vi "svx_Oct_Waterfall Init.vi"(3 "Container State":T5, 4 "Previous State":variant=variant(cluster{"X Scale Width %":dbl, "Y Scale Height %":dbl, "X-Axis Range":cluster{"Minimum":dbl, "Maximum":dbl}, "Y-Axis Range":cluster{"Minimum":dbl, "Maximum":dbl}, "Z-Axis Range":cluster{"Minimum":dbl, "Maximum":dbl}, "# Plots Updated":i32, "Plot Color":u32, "Frame Color":u32, "Background Color":u32, "Property Name":string, "Just Loaded?":bool, "Initial AutoScale Y":bool, "AutoScale X":u8, "AutoScale Y":u8, "AutoScale Z":u8, "Plot Transparency":bool, "X-Axis Name":string, "Y-Axis Name":string, "Z-Axis Name":string, "X-Axis Scaling Factor":cluster{"Offset":dbl, "Multiplier":dbl}, "Y-Axis Scaling Factor":cluster{"Offset":dbl, "Multiplier":dbl}, "Z-Axis Scaling Factor":cluster{"Offset":dbl, "Multiplier":dbl}, "X-Scale Visible":bool, "Y-Scale Visible":bool, "Z-Scale Visible":bool, "X-Scale Label Visible":bool, "Y-Scale Label Visible":bool, "Z-Scale Label Visible":bool, "X-Axis Range Scaled":cluster{"Minimum":dbl, "Maximum":dbl}, "Y-Axis Range Scaled":cluster{"Minimum":dbl, "Maximum":dbl}, "Z-Axis Range Scaled":cluster{"Minimum":dbl, "Maximum":dbl}, "Rev Z Order":bool, "First Time Ever":bool} {"X Scale Width %"=0.0, "Y Scale Height %"=0.0, "X-Axis Range"={"Minimum"=0.0, "Maximum"=0.0}, "Y-Axis Range"={"Minimum"=0.0, "Maximum"=0.0}, "Z-Axis Range"={"Minimum"=0.0, "Maximum"=0.0}, "# Plots Updated"=0, "Plot Color"=0, "Frame Color"=0, "Background Color"=0, "Property Name"="", "Just Loaded?"=FALSE, "Initial AutoScale Y"=FALSE, "AutoScale X"=0, "AutoScale Y"=0, "AutoScale Z"=0, "Plot Transparency"=FALSE, "X-Axis Name"="", "Y-Axis Name"="", "Z-Axis Name"="", "X-Axis Scaling Factor"={"Offset"=0.0, "Multiplier"=0.0}, "Y-Axis Scaling Factor"={"Offset"=0.0, "Multiplier"=0.0}, "Z-Axis Scaling Factor"={"Offset"=0.0, "Multiplier"=0.0}, "X-Scale Visible"=FALSE, "Y-Scale Visible"=FALSE, "Z-Scale Visible"=FALSE, "X-Scale Label Visible"=FALSE, "Y-Scale Label Visible"=FALSE, "Z-Scale Label Visible"=FALSE, "X-Axis Range Scaled"={"Minimum"=0.0, "Maximum"=0.0}, "Y-Axis Range Scaled"={"Minimum"=0.0, "Maximum"=0.0}, "Z-Axis Range Scaled"={"Minimum"=0.0, "Maximum"=0.0}, "Rev Z Order"=FALSE, "First Time Ever"=FALSE}), 5 "Previous Version":T4) -> (2 "Current State":T3={"X Scale Width %"=50.0, "Y Scale Height %"=50.0, "X-Axis Range"={"Minimum"=0.0, "Maximum"=10.0}, "Y-Axis Range"={"Minimum"=0.0, "Maximum"=10.0}, "Z-Axis Range"={"Minimum"=0.0, "Maximum"=10.0}, "Plot Color"=0, "Frame Color"=61212, "Background Color"=16252785, "Initial AutoScale Y"=TRUE, "AutoScale X"=2, "AutoScale Y"=2, "AutoScale Z"=2, "Plot Transparency"=FALSE, "X-Axis Name"="Frequency", "Y-Axis Name"="Amplitude", "Z-Axis Name"="", "X-Axis Scaling Factor"={"Offset"=0.0, "Multiplier"=1.0}, "Y-Axis Scaling Factor"={"Offset"=0.0, "Multiplier"=1.0}, "Z-Axis Scaling Factor"={"Offset"=0.0, "Multiplier"=1.0}, "X-Scale Visible"=TRUE, "Y-Scale Visible"=TRUE, "Z-Scale Visible"=TRUE, "X-Scale Label Visible"=TRUE, "Y-Scale Label Visible"=TRUE, "Z-Scale Label Visible"=TRUE, "X-Axis Range Scaled"={"Minimum"=0.0, "Maximum"=10.0}, "Y-Axis Range Scaled"={"Minimum"=0.0, "Maximum"=10.0}, "Z-Axis Range Scaled"={"Minimum"=0.0, "Maximum"=10.0}, "Rev Z Order"=FALSE, "X-Scale Format Str"="%#.4g", "Y-Scale Format Str"="%#.4g", "Z-Scale Format Str"="%#.4g", "Decor color"=12369084, "Scale Range Change"=refnum, "out of state queue"=refnum, "property nodes"=refnum})   [LabVIEW 2017, in "SVX Octave Waterfall Graph.xctl"]
uses:
  <vilib>/addons/_XControls/Octave Waterfall Graph/SVX Octave Waterfall Graph.xctl
  <vilib>/addons/_XControls/Octave Waterfall Graph/subVIs/svx_Oct_Waterfall State.ctl
  <vilib>/_xctls/Container State.ctl
  <vilib>/_xctls/Version.ctl
  <vilib>/_xctls/XControlSupport.lvlib
panel:
  out "background":bool
  in  "Indicator State (6.0.0.0, 7.0.0.0)":T1={"X Scale Width %"=80.0, "Y Scale Height %"=40.0, "X-Axis Range"={"Minimum"=0.0, "Maximum"=10.0}, "Y-Axis Range"={"Minimum"=0.0, "Maximum"=10.0}, "Z-Axis Range"={"Minimum"=0.0, "Maximum"=10.0}, "# Plots Updated"=0, "Plot Color"=61212, "Frame Color"=16252785, "Background Color"=16777222, "Property Name"=[], "Just Loaded?"=TRUE, "Initial AutoScale Y"=TRUE, "AutoScale X"=2, "AutoScale Y"=2, "AutoScale Z"=2, "Plot Transparency"=FALSE, "X-Axis Name"="Frequency", "Y-Axis Name"="Amplitude", "Z-Axis Name"="", "X-Axis Scaling Factor"={"Offset"=0.0, "Multiplier"=1.0}, "Y-Axis Scaling Factor"={"Offset"=0.0, "Multiplier"=1.0}, "Z-Axis Scaling Factor"={"Offset"=0.0, "Multiplier"=1.0}, "X-Scale Visible"=TRUE, "Y-Scale Visible"=TRUE, "Z-Scale Visible"=TRUE, "X-Scale Label Visible"=TRUE, "Y-Scale Label Visible"=TRUE, "Z-Scale Label Visible"=TRUE, "X-Axis Range Scaled"={"Minimum"=0.0, "Maximum"=10.0}, "Y-Axis Range Scaled"={"Minimum"=0.0, "Maximum"=10.0}, "Z-Axis Range Scaled"={"Minimum"=0.0, "Maximum"=10.0}, "Rev Z Order"=FALSE, "First Time Ever"=TRUE, "X-Scale Format Str"="%#.4g", "Y-Scale Format Str"="%#.4g", "Z-Scale Format Str"="%#.4g", "Decor color"=12369084, "Facade VI"=refnum, "Scale Range Change"=refnum}
  in  "Indicator State (5.0.0.0)":T2={"X Scale Width %"=80.0, "Y Scale Height %"=40.0, "X-Axis Range"={"Minimum"=0.0, "Maximum"=10.0}, "Y-Axis Range"={"Minimum"=0.0, "Maximum"=10.0}, "Z-Axis Range"={"Minimum"=0.0, "Maximum"=10.0}, "# Plots Updated"=0, "Plot Color"=61212, "Frame Color"=16252785, "Background Color"=16777222, "Property Name"=[], "Just Loaded?"=TRUE, "Initial AutoScale Y"=TRUE, "AutoScale X"=2, "AutoScale Y"=2, "AutoScale Z"=2, "Plot Transparency"=FALSE, "X-Axis Name"="Frequency", "Y-Axis Name"="Amplitude", "Z-Axis Name"="", "X-Axis Scaling Factor"={"Offset"=0.0, "Multiplier"=1.0}, "Y-Axis Scaling Factor"={"Offset"=0.0, "Multiplier"=1.0}, "Z-Axis Scaling Factor"={"Offset"=0.0, "Multiplier"=1.0}, "X-Scale Visible"=TRUE, "Y-Scale Visible"=TRUE, "Z-Scale Visible"=TRUE, "X-Scale Label Visible"=TRUE, "Y-Scale Label Visible"=TRUE, "Z-Scale Label Visible"=TRUE, "X-Axis Range Scaled"={"Minimum"=0.0, "Maximum"=10.0}, "Y-Axis Range Scaled"={"Minimum"=0.0, "Maximum"=10.0}, "Z-Axis Range Scaled"={"Minimum"=0.0, "Maximum"=10.0}, "Rev Z Order"=FALSE, "First Time Ever"=TRUE, "X-Scale Format Str"="%#.4g", "Y-Scale Format Str"="%#.4g", "Z-Scale Format Str"="%#.4g", "Decor color"=12369084, "Facade VI"=refnum}
  in  "Default Indicator State":T3={"X Scale Width %"=80.0, "Y Scale Height %"=40.0, "X-Axis Range"={"Minimum"=0.0, "Maximum"=10.0}, "Y-Axis Range"={"Minimum"=0.0, "Maximum"=10.0}, "Z-Axis Range"={"Minimum"=0.0, "Maximum"=10.0}, "Plot Color"=6618880, "Frame Color"=16252785, "Background Color"=16777222, "Initial AutoScale Y"=TRUE, "AutoScale X"=2, "AutoScale Y"=2, "AutoScale Z"=2, "Plot Transparency"=FALSE, "X-Axis Name"="Frequency", "Y-Axis Name"="Amplitude", "Z-Axis Name"="", "X-Axis Scaling Factor"={"Offset"=0.0, "Multiplier"=1.0}, "Y-Axis Scaling Factor"={"Offset"=0.0, "Multiplier"=1.0}, "Z-Axis Scaling Factor"={"Offset"=0.0, "Multiplier"=1.0}, "X-Scale Visible"=TRUE, "Y-Scale Visible"=TRUE, "Z-Scale Visible"=TRUE, "X-Scale Label Visible"=TRUE, "Y-Scale Label Visible"=TRUE, "Z-Scale Label Visible"=TRUE, "X-Axis Range Scaled"={"Minimum"=0.0, "Maximum"=10.0}, "Y-Axis Range Scaled"={"Minimum"=0.0, "Maximum"=10.0}, "Z-Axis Range Scaled"={"Minimum"=0.0, "Maximum"=10.0}, "Rev Z Order"=FALSE, "X-Scale Format Str"="%#.4g", "Y-Scale Format Str"="%#.4g", "Z-Scale Format Str"="%#.4g", "Decor color"=12369084, "Scale Range Change"=refnum, "out of state queue"=refnum, "property nodes"=refnum}
  in  "Default Control State":T3={"X Scale Width %"=80.0, "Y Scale Height %"=40.0, "X-Axis Range"={"Minimum"=0.0, "Maximum"=10.0}, "Y-Axis Range"={"Minimum"=0.0, "Maximum"=10.0}, "Z-Axis Range"={"Minimum"=0.0, "Maximum"=10.0}, "Plot Color"=6618880, "Frame Color"=16252785, "Background Color"=16777222, "Initial AutoScale Y"=TRUE, "AutoScale X"=2, "AutoScale Y"=2, "AutoScale Z"=2, "Plot Transparency"=FALSE, "X-Axis Name"="Frequency", "Y-Axis Name"="Amplitude", "Z-Axis Name"="", "X-Axis Scaling Factor"={"Offset"=0.0, "Multiplier"=1.0}, "Y-Axis Scaling Factor"={"Offset"=0.0, "Multiplier"=1.0}, "Z-Axis Scaling Factor"={"Offset"=0.0, "Multiplier"=1.0}, "X-Scale Visible"=TRUE, "Y-Scale Visible"=TRUE, "Z-Scale Visible"=TRUE, "X-Scale Label Visible"=TRUE, "Y-Scale Label Visible"=TRUE, "Z-Scale Label Visible"=TRUE, "X-Axis Range Scaled"={"Minimum"=0.0, "Maximum"=10.0}, "Y-Axis Range Scaled"={"Minimum"=0.0, "Maximum"=10.0}, "Z-Axis Range Scaled"={"Minimum"=0.0, "Maximum"=10.0}, "Rev Z Order"=FALSE, "X-Scale Format Str"="%#.4g", "Y-Scale Format Str"="%#.4g", "Z-Scale Format Str"="%#.4g", "Decor color"=12369084, "Scale Range Change"=refnum, "out of state queue"=refnum, "property nodes"=refnum}
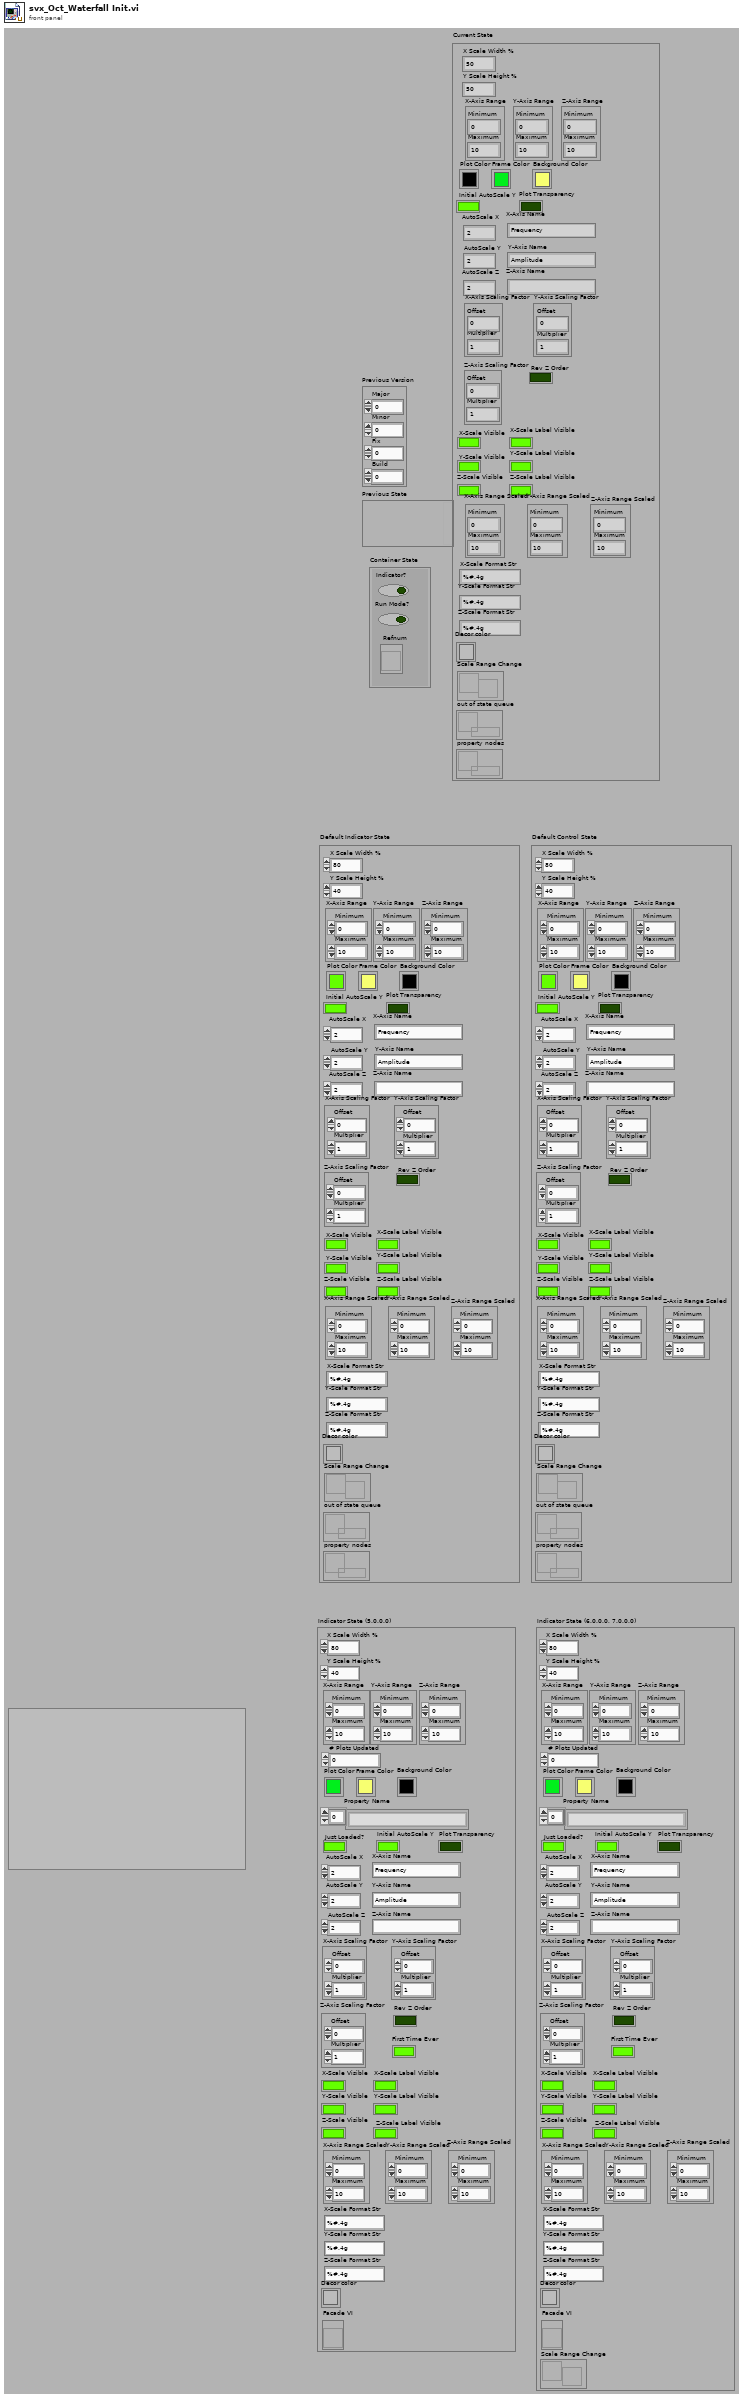
[diagram p1: front panel]
types:
  T1 = cluster{"X Scale Width %":dbl, "Y Scale Height %":dbl, "X-Axis Range":cluster{"Minimum":dbl, "Maximum":dbl}, "Y-Axis Range":cluster{"Minimum":dbl, "Maximum":dbl}, "Z-Axis Range":cluster{"Minimum":dbl, "Maximum":dbl}, "# Plots Updated":i32, "Plot Color":u32, "Frame Color":u32, "Background Color":u32, "Property Name":string[], "Just Loaded?":bool, "Initial AutoScale Y":bool, "AutoScale X":u8, "AutoScale Y":u8, "AutoScale Z":u8, "Plot Transparency":bool, "X-Axis Name":string, "Y-Axis Name":string, "Z-Axis Name":string, "X-Axis Scaling Factor":cluster{"Offset":dbl, "Multiplier":dbl}, "Y-Axis Scaling Factor":cluster{"Offset":dbl, "Multiplier":dbl}, "Z-Axis Scaling Factor":cluster{"Offset":dbl, "Multiplier":dbl}, "X-Scale Visible":bool, "Y-Scale Visible":bool, "Z-Scale Visible":bool, "X-Scale Label Visible":bool, "Y-Scale Label Visible":bool, "Z-Scale Label Visible":bool, "X-Axis Range Scaled":cluster{"Minimum":dbl, "Maximum":dbl}, "Y-Axis Range Scaled":cluster{"Minimum":dbl, "Maximum":dbl}, "Z-Axis Range Scaled":cluster{"Minimum":dbl, "Maximum":dbl}, "Rev Z Order":bool, "First Time Ever":bool, "X-Scale Format Str":string, "Y-Scale Format Str":string, "Z-Scale Format Str":string, "Decor color":u32, "Facade VI":refnum<vi>, "Scale Range Change":refnum<user-event>}
  T2 = cluster{"X Scale Width %":dbl, "Y Scale Height %":dbl, "X-Axis Range":cluster{"Minimum":dbl, "Maximum":dbl}, "Y-Axis Range":cluster{"Minimum":dbl, "Maximum":dbl}, "Z-Axis Range":cluster{"Minimum":dbl, "Maximum":dbl}, "# Plots Updated":i32, "Plot Color":u32, "Frame Color":u32, "Background Color":u32, "Property Name":string[], "Just Loaded?":bool, "Initial AutoScale Y":bool, "AutoScale X":u8, "AutoScale Y":u8, "AutoScale Z":u8, "Plot Transparency":bool, "X-Axis Name":string, "Y-Axis Name":string, "Z-Axis Name":string, "X-Axis Scaling Factor":cluster{"Offset":dbl, "Multiplier":dbl}, "Y-Axis Scaling Factor":cluster{"Offset":dbl, "Multiplier":dbl}, "Z-Axis Scaling Factor":cluster{"Offset":dbl, "Multiplier":dbl}, "X-Scale Visible":bool, "Y-Scale Visible":bool, "Z-Scale Visible":bool, "X-Scale Label Visible":bool, "Y-Scale Label Visible":bool, "Z-Scale Label Visible":bool, "X-Axis Range Scaled":cluster{"Minimum":dbl, "Maximum":dbl}, "Y-Axis Range Scaled":cluster{"Minimum":dbl, "Maximum":dbl}, "Z-Axis Range Scaled":cluster{"Minimum":dbl, "Maximum":dbl}, "Rev Z Order":bool, "First Time Ever":bool, "X-Scale Format Str":string, "Y-Scale Format Str":string, "Z-Scale Format Str":string, "Decor color":u32, "Facade VI":refnum<vi>}
  T3 = typedef "SVX Octave Waterfall Graph.xctl/svx_Oct_Waterfall State.ctl" = cluster{"X Scale Width %":dbl, "Y Scale Height %":dbl, "X-Axis Range":cluster{"Minimum":dbl, "Maximum":dbl}, "Y-Axis Range":cluster{"Minimum":dbl, "Maximum":dbl}, "Z-Axis Range":cluster{"Minimum":dbl, "Maximum":dbl}, "Plot Color":u32, "Frame Color":u32, "Background Color":u32, "Initial AutoScale Y":bool, "AutoScale X":u8, "AutoScale Y":u8, "AutoScale Z":u8, "Plot Transparency":bool, "X-Axis Name":string, "Y-Axis Name":string, "Z-Axis Name":string, "X-Axis Scaling Factor":cluster{"Offset":dbl, "Multiplier":dbl}, "Y-Axis Scaling Factor":cluster{"Offset":dbl, "Multiplier":dbl}, "Z-Axis Scaling Factor":cluster{"Offset":dbl, "Multiplier":dbl}, "X-Scale Visible":bool, "Y-Scale Visible":bool, "Z-Scale Visible":bool, "X-Scale Label Visible":bool, "Y-Scale Label Visible":bool, "Z-Scale Label Visible":bool, "X-Axis Range Scaled":cluster{"Minimum":dbl, "Maximum":dbl}, "Y-Axis Range Scaled":cluster{"Minimum":dbl, "Maximum":dbl}, "Z-Axis Range Scaled":cluster{"Minimum":dbl, "Maximum":dbl}, "Rev Z Order":bool, "X-Scale Format Str":string, "Y-Scale Format Str":string, "Z-Scale Format Str":string, "Decor color":u32, "Scale Range Change":refnum<user-event>, "out of state queue":refnum<queue>, "property nodes":refnum<queue>}
  T4 = typedef "XControlSupport.lvlib/Version.ctl" = cluster{"Major":u16, "Minor":u16, "Fix":u16, "Build":u16}
  T5 = typedef "XControlSupport.lvlib/Container State.ctl" = cluster{"Indicator?":bool, "Run Mode?":bool, " Refnum":refnum<vi>}
  T6 = cluster{"Minimum":dbl, "Maximum":dbl, "Kind":enum16{"X-Scale", "Y-Scale", "Z-Scale"}}
  T7 = cluster{"use queue?":bool, "X-Axis Range":cluster{"Minimum":dbl, "Maximum":dbl}, "Y-Axis Range":cluster{"Minimum":dbl, "Maximum":dbl}, "Z-Axis Range":cluster{"Minimum":dbl, "Maximum":dbl}, "X-Axis Range Scaled":cluster{"Minimum":dbl, "Maximum":dbl}, "Y-Axis Range Scaled":cluster{"Minimum":dbl, "Maximum":dbl}, "Z-Axis Range Scaled":cluster{"Minimum":dbl, "Maximum":dbl}, "AutoScale X":u8, "AutoScale Y":u8, "AutoScale Z":u8, "background":refnum<vi>}
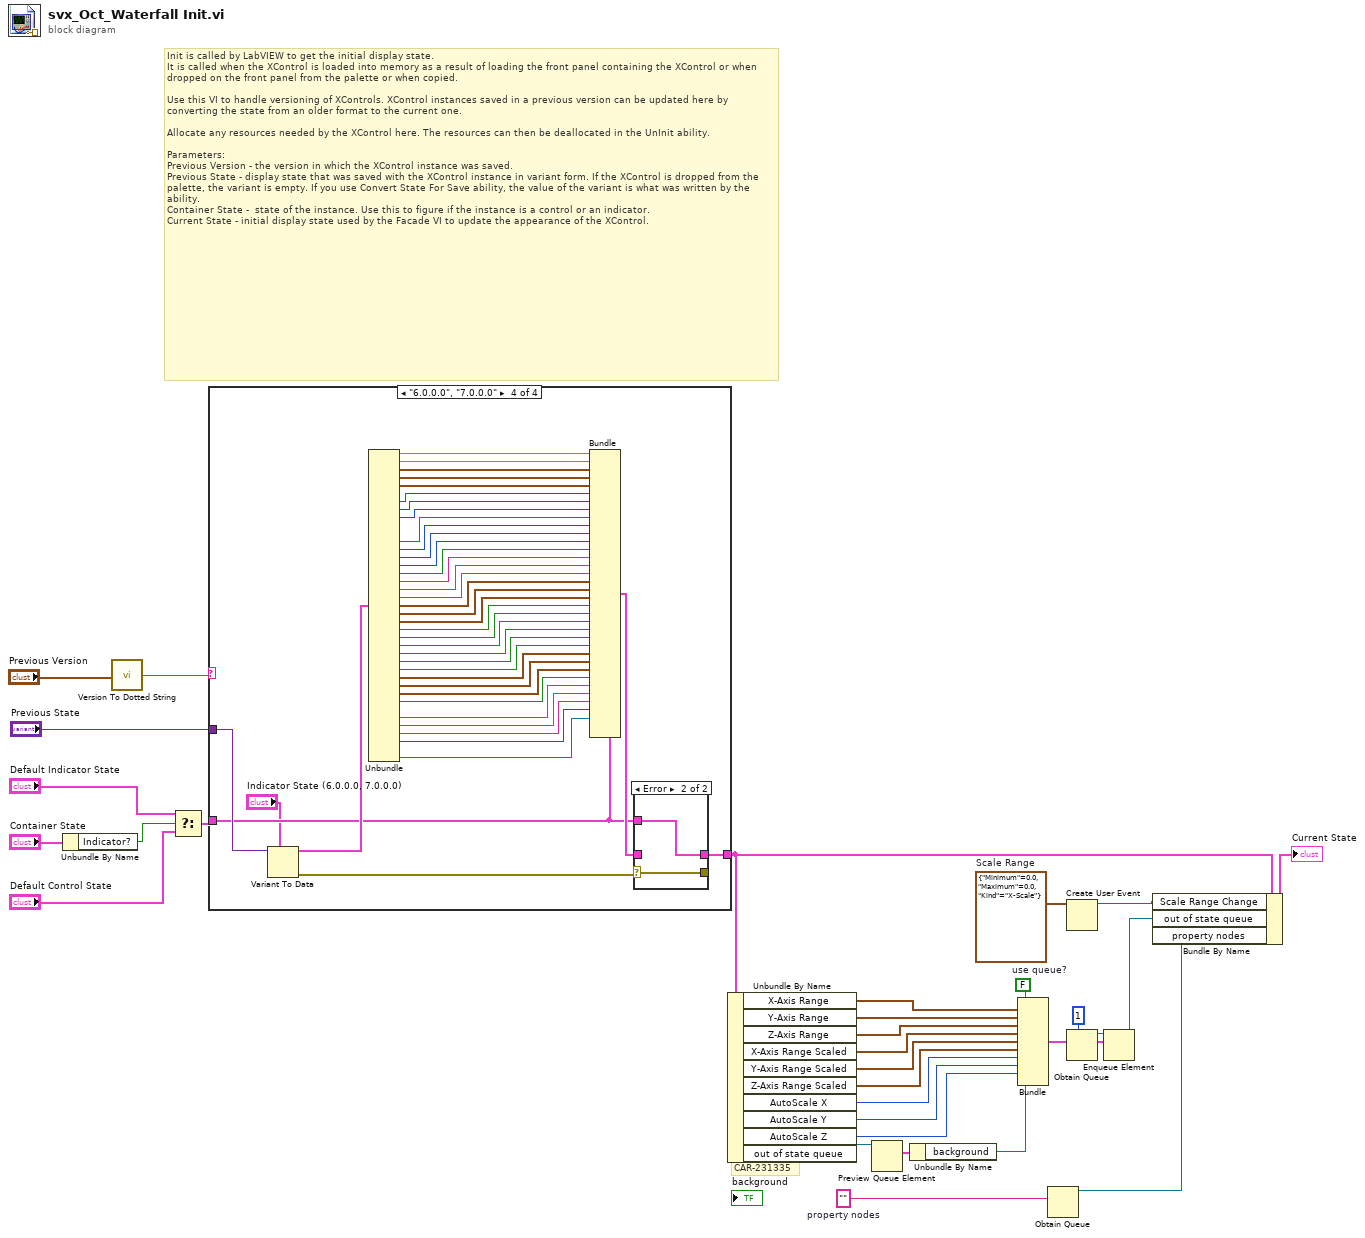
[diagram p0: block diagram]
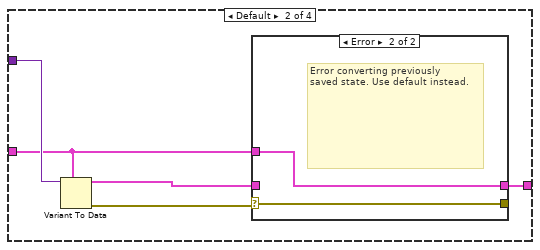
[diagram p3: hidden frame]
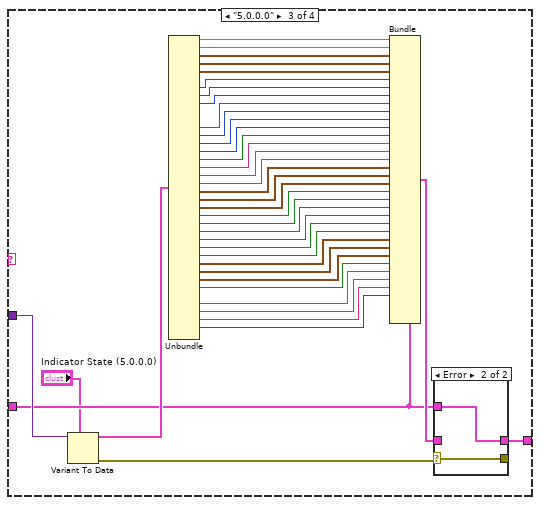
[diagram p5: hidden frame]
diagram:
  w7 = ""  # property nodes
  w15 = FALSE  # use queue?
  w23 = T6 {"Minimum"=0.0, "Maximum"=0.0, "Kind"=enum."X-Scale"}  # Scale Range
  # "CAR-231335"
  # "Init is called by LabVIEW to get the initial display state.\nIt is called when the XControl is loaded into memory as a result of loading the front panel containing the XControl or when dropped on the front panel from the palette or when copied.\n\nUse this VI to handle versioning of XControls. XControl instances saved in a previous version can be updated here by converting the state from an older format to the current one.\n\nAllocate any resources needed by the XControl here. The resources can then be deallocated in the UnInit ability.\n\nParameters:\nPrevious Version - the version in which the XControl instance was saved.\nPrevious State - display state that was saved with the XControl instance in variant form. If the XControl is dropped from the palette, the variant is empty. If you use Convert State For Save ability, the value of the variant is what was written by the ability. \nContainer State -  state of the instance. Use this to figure if the instance is a control or an indicator.\nCurrent State - initial display state used by the Facade VI to update the appearance of the XControl."
  n1 = Unbundle By Name("Container State") -> ("Indicator?"=w29:bool)
  n2 = call <vilib>:"Version To Dotted String.vi"("Version"="Previous Version") -> ("String Version"=w24:string)
  n3 = Select(t="Default Indicator State", s=w29, f="Default Control State") -> (s? t:f=w28:T3)
  n4 = case shown="\"6.0.0.0\", \"7.0.0.0\"" w24 {
    tunnel: "Previous State" -> [_ w37 w73 w118]
    tunnel: [w32 w34 w70 w116] -> w6
    tunnel: w28 -> [w32 w35 w72 w117]
    frame "0.0.0.0" {
      # "Just created, use default state"
    }
    frame Default {
      n5 = Variant To Data(type=w35, Variant=w37) -> (data=w33:T3, error out=w36:errorcluster)  [unwired: 1 in]
      n6 = case shown="Error" w36 {
        selector: w36 -> [w39 w40]
        tunnel: w33 -> [w38 _]
        tunnel: [w38 w41] -> w34
        tunnel: w35 -> [_ w41]
        tunnel: [w39 w40] -> _
        frame No Error {
        }
        frame Error {
          # "Error converting previously \nsaved state. Use default instead."
        }
      }
    }
    frame "5.0.0.0" {
      n7 = Variant To Data(type="Indicator State (5.0.0.0)", Variant=w73) -> (data=w75:T2, error out=w74:errorcluster)  [unwired: 1 in]
      n8 = Unbundle(w75) -> ("X Scale Width %"=w76:dbl, "Y Scale Height %"=w77:dbl, "X-Axis Range"=w78:cluster{"Minimum":dbl, "Maximum":dbl}, "Y-Axis Range"=w79:cluster{"Minimum":dbl, "Maximum":dbl}, "Z-Axis Range"=w80:cluster{"Minimum":dbl, "Maximum":dbl}, "Plot Color"=w69:u32, "Frame Color"=w68:u32, "Background Color"=w67:u32, "Initial AutoScale Y"=w66:bool, "AutoScale X"=w65:u8, "AutoScale Y"=w64:u8, "AutoScale Z"=w63:u8, "Plot Transparency"=w62:bool, "X-Axis Name"=w61:string, "Y-Axis Name"=w60:string, "Z-Axis Name"=w59:string, "X-Axis Scaling Factor"=w58:cluster{"Offset":dbl, "Multiplier":dbl}, "Y-Axis Scaling Factor"=w57:cluster{"Offset":dbl, "Multiplier":dbl}, "Z-Axis Scaling Factor"=w56:cluster{"Offset":dbl, "Multiplier":dbl}, "X-Scale Visible"=w55:bool, "Y-Scale Visible"=w54:bool, "Z-Scale Visible"=w53:bool, "X-Scale Label Visible"=w52:bool, "Y-Scale Label Visible"=w51:bool, "Z-Scale Label Visible"=w50:bool, "X-Axis Range Scaled"=w49:cluster{"Minimum":dbl, "Maximum":dbl}, "Y-Axis Range Scaled"=w48:cluster{"Minimum":dbl, "Maximum":dbl}, "Z-Axis Range Scaled"=w47:cluster{"Minimum":dbl, "Maximum":dbl}, "Rev Z Order"=w46:bool, "X-Scale Format Str"=w45:string, "Y-Scale Format Str"=w44:string, "Z-Scale Format Str"=w43:string, "Decor color"=w42:u32)  [unwired: 5 out]
      n9 = Bundle(cluster=w72, "X Scale Width %"=w76, "Y Scale Height %"=w77, "X-Axis Range"=w78, "Y-Axis Range"=w79, "Z-Axis Range"=w80, "Plot Color"=w69, "Frame Color"=w68, "Background Color"=w67, "Initial AutoScale Y"=w66, "AutoScale X"=w65, "AutoScale Y"=w64, "AutoScale Z"=w63, "Plot Transparency"=w62, "X-Axis Name"=w61, "Y-Axis Name"=w60, "Z-Axis Name"=w59, "X-Axis Scaling Factor"=w58, "Y-Axis Scaling Factor"=w57, "Z-Axis Scaling Factor"=w56, "X-Scale Visible"=w55, "Y-Scale Visible"=w54, "Z-Scale Visible"=w53, "X-Scale Label Visible"=w52, "Y-Scale Label Visible"=w51, "Z-Scale Label Visible"=w50, "X-Axis Range Scaled"=w49, "Y-Axis Range Scaled"=w48, "Z-Axis Range Scaled"=w47, "Rev Z Order"=w46, "X-Scale Format Str"=w45, "Y-Scale Format Str"=w44, "Z-Scale Format Str"=w43, "Decor color"=w42) -> (w81:T3)  [unwired: 3 in]
      n10 = case shown="Error" w74 {
        selector: w74 -> [w83 w84]
        tunnel: w81 -> [w82 _]
        tunnel: [w82 w85] -> w70
        tunnel: w72 -> [_ w85]
        tunnel: [w83 w84] -> _
        frame No Error {
        }
        frame Error {
        }
      }
    }
    frame "6.0.0.0", "7.0.0.0" {
      n11 = Variant To Data(type="Indicator State (6.0.0.0, 7.0.0.0)", Variant=w118) -> (data=w120:T1, error out=w119:errorcluster)  [unwired: 1 in]
      n12 = Unbundle(w120) -> ("X Scale Width %"=w121:dbl, "Y Scale Height %"=w122:dbl, "X-Axis Range"=w123:cluster{"Minimum":dbl, "Maximum":dbl}, "Y-Axis Range"=w124:cluster{"Minimum":dbl, "Maximum":dbl}, "Z-Axis Range"=w125:cluster{"Minimum":dbl, "Maximum":dbl}, "Plot Color"=w115:u32, "Frame Color"=w114:u32, "Background Color"=w113:u32, "Initial AutoScale Y"=w112:bool, "AutoScale X"=w111:u8, "AutoScale Y"=w110:u8, "AutoScale Z"=w109:u8, "Plot Transparency"=w108:bool, "X-Axis Name"=w107:string, "Y-Axis Name"=w106:string, "Z-Axis Name"=w105:string, "X-Axis Scaling Factor"=w104:cluster{"Offset":dbl, "Multiplier":dbl}, "Y-Axis Scaling Factor"=w103:cluster{"Offset":dbl, "Multiplier":dbl}, "Z-Axis Scaling Factor"=w102:cluster{"Offset":dbl, "Multiplier":dbl}, "X-Scale Visible"=w101:bool, "Y-Scale Visible"=w100:bool, "Z-Scale Visible"=w99:bool, "X-Scale Label Visible"=w98:bool, "Y-Scale Label Visible"=w97:bool, "Z-Scale Label Visible"=w96:bool, "X-Axis Range Scaled"=w95:cluster{"Minimum":dbl, "Maximum":dbl}, "Y-Axis Range Scaled"=w94:cluster{"Minimum":dbl, "Maximum":dbl}, "Z-Axis Range Scaled"=w93:cluster{"Minimum":dbl, "Maximum":dbl}, "Rev Z Order"=w92:bool, "X-Scale Format Str"=w91:string, "Y-Scale Format Str"=w90:string, "Z-Scale Format Str"=w89:string, "Decor color"=w88:u32, "Scale Range Change"=w86:refnum<user-event>)  [unwired: 5 out]
      n13 = Bundle(cluster=w117, "X Scale Width %"=w121, "Y Scale Height %"=w122, "X-Axis Range"=w123, "Y-Axis Range"=w124, "Z-Axis Range"=w125, "Plot Color"=w115, "Frame Color"=w114, "Background Color"=w113, "Initial AutoScale Y"=w112, "AutoScale X"=w111, "AutoScale Y"=w110, "AutoScale Z"=w109, "Plot Transparency"=w108, "X-Axis Name"=w107, "Y-Axis Name"=w106, "Z-Axis Name"=w105, "X-Axis Scaling Factor"=w104, "Y-Axis Scaling Factor"=w103, "Z-Axis Scaling Factor"=w102, "X-Scale Visible"=w101, "Y-Scale Visible"=w100, "Z-Scale Visible"=w99, "X-Scale Label Visible"=w98, "Y-Scale Label Visible"=w97, "Z-Scale Label Visible"=w96, "X-Axis Range Scaled"=w95, "Y-Axis Range Scaled"=w94, "Z-Axis Range Scaled"=w93, "Rev Z Order"=w92, "X-Scale Format Str"=w91, "Y-Scale Format Str"=w90, "Z-Scale Format Str"=w89, "Decor color"=w88, "Scale Range Change"=w86) -> (w126:T3)  [unwired: 2 in]
      n14 = case shown="Error" w119 {
        selector: w119 -> [w128 w129]
        tunnel: w126 -> [w127 _]
        tunnel: [w127 w130] -> w116
        tunnel: w117 -> [_ w130]
        tunnel: [w128 w129] -> _
        frame No Error {
        }
        frame Error {
        }
      }
    }
  }
  n15 = Unbundle By Name(w6) -> ("X-Axis Range"=w17:cluster{"Minimum":dbl, "Maximum":dbl}, "Y-Axis Range"=w16:cluster{"Minimum":dbl, "Maximum":dbl}, "Z-Axis Range"=w12:cluster{"Minimum":dbl, "Maximum":dbl}, "X-Axis Range Scaled"=w11:cluster{"Minimum":dbl, "Maximum":dbl}, "Y-Axis Range Scaled"=w10:cluster{"Minimum":dbl, "Maximum":dbl}, "Z-Axis Range Scaled"=w9:cluster{"Minimum":dbl, "Maximum":dbl}, "AutoScale X"=w18:u8, "AutoScale Y"=w19:u8, "AutoScale Z"=w20:u8, "out of state queue"=w2:refnum<queue>)
  n16 = Preview Queue Element(queue=w2) -> (element=w3:T7)  [unwired: 2 in, 3 out]
  n17 = Unbundle By Name(w3) -> ("background"=w1:refnum<vi>)
  n18 = Bundle("use queue?"=w15, "X-Axis Range"=w17, "Y-Axis Range"=w16, "Z-Axis Range"=w12, "X-Axis Range Scaled"=w11, "Y-Axis Range Scaled"=w10, "Z-Axis Range Scaled"=w9, "AutoScale X"=w18, "AutoScale Y"=w19, "AutoScale Z"=w20, "background"=w1) -> (w13:T7)  [unwired: 1 in]
  n19 = Obtain Queue(element data type=w7) -> (queue out=w4:refnum<queue>)  [unwired: 4 in, 2 out]
  n20 = Create User Event(user event datatype=w23) -> (user event=w22:refnum<user-event>)  [unwired: 1 in, 1 out]
  n21 = Obtain Queue(max queue size (-1, unlimited)=1, element data type=w13) -> (queue out=w8:refnum<queue>)  [unwired: 3 in, 2 out]
  n22 = Enqueue Element(queue=w8, element=w13) -> (queue out=w5:refnum<queue>)  [unwired: 2 in, 2 out]
  n23 = Bundle By Name(cluster=w6, "Scale Range Change"=w22, "out of state queue"=w5, "property nodes"=w4) -> (→"Current State":T3)
